vi "Draw Overlay.vi"(8 "error in (no error)":errorcluster, 11 "Terminal in":refnum<class "Terminal.lvclass">) -> (0 "error out":errorcluster, 3 "Terminal out":refnum<class "Terminal.lvclass">)   [LabVIEW 2020, in "Terminal.lvlib" / "Terminal.lvclass"]
uses:
  Terminal.lvclass
  Text Attributes.ctl
  Terminal.lvclass/Terminal.ctl
  <vilib>/IlluminatedG/lv-stream/Connection/Connection.lvclass
  Terminal.lvlib
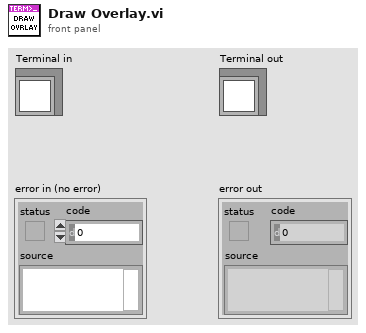
[diagram p1: front panel]
types:
  T1 = typedef "Terminal.lvlib/Text Attributes.ctl" = cluster{"FG":u32, "BG":u32, "Bold":bool, "Italic":bool, "Underline":bool, "Strike":bool, "Inverse":bool}
  T2 = typedef "Terminal.lvlib/Terminal.lvclass/Ref Data.ctl" = cluster{"Connection":refnum<class "Connection.lvclass">, "Read Loop Running":bool, "Parse State":T3, "Terminal Options":T7, "Font Metrics":T10, "Scroll":i32, "Close Read Loop":bool}
  T3 = typedef "Terminal.lvlib/Terminal.lvclass/Parse State.ctl" = cluster{"Buffer State":T4, "Cursor":T5, "Attributes":T1}
  T4 = typedef "Terminal.lvlib/Terminal.lvclass/Buffer State.ctl" = cluster{"Sequence":string, "ESC":bool, "Alt Buf":bool}
  T5 = typedef "Terminal.lvlib/Terminal.lvclass/Cursor.ctl" = cluster{"Cur":T6, "Saved":T6}
  T6 = typedef "Terminal.lvlib/Terminal.lvclass/Position.ctl" = cluster{"Row":i32, "Col":i32}
  T7 = typedef "Terminal.lvlib/Terminal Options.ctl" = cluster{"Implied CR with LF":bool, "Local Echo":bool, "Tab Width":i32, "Color Scheme":T8, "Default FG":T9, "Default BG":T9, "History Length":i32, "Font Face":string, "Font Size":i16, "Rows":i32, "Cols":i32}
  T8 = typedef "Terminal.lvlib/Color Scheme.ctl" = cluster{"Black":u32, "Red":u32, "Green":u32, "Yellow":u32, "Blue":u32, "Magenta":u32, "Cyan":u32, "White":u32, "Bright Black":u32, "Bright Red":u32, "Bright Green":u32, "Bright Yellow":u32, "Bright Blue":u32, "Bright Magenta":u32, "Bright Cyan":u32, "Bright White":u32}
  T9 = typedef "Terminal.lvlib/Color.ctl" = i8
  T10 = typedef "Terminal.lvlib/Terminal.lvclass/Font Metrics.ctl" = cluster{"Width":i16, "Height":i16}
  T11 = typedef "LVBoundsTypeDef.ctl" = cluster{"Width":u32, "Height":u32}
  T12 = cluster{"Font Name:":string, "Size":i16, "Strikeout?":bool, "Italic?":bool, "Underline?":bool, "Outline?":bool, "Shadow?":bool, "Bold?":bool}
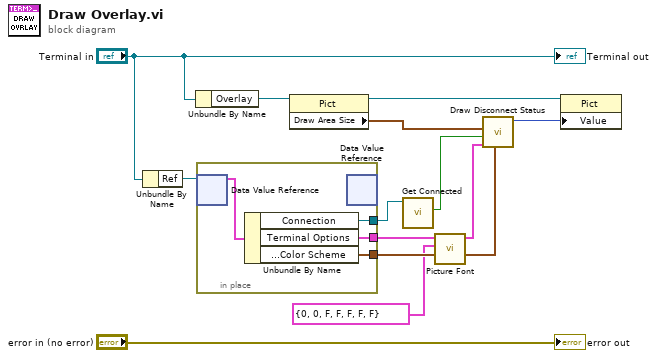
[diagram p0: block diagram]
diagram:
  n1 = Unbundle By Name("Terminal in") -> ("Ref"=w11:refnum<data-value>)
  n2 = Unbundle By Name("Terminal in") -> ("Overlay"=w12:refnum<vi>)
  n3 = in-place {
    in-place-border: [w16] -> w9
    in-place-border: [w15] -> w4
    in-place-border: [w14] -> w3
    n4 = in-place-dvr #1(w11) -> (w17:T2)  [unwired: 1 out]
    n5 = Unbundle By Name(w17) -> ("Connection"=w16:refnum<class "Connection.lvclass">, "Terminal Options"=w14:T7, "Terminal Options.Color Scheme"=w15:T8)
    n6 = in-place-dvr #1() -> ()  [unwired: 1 in, 2 out]
  }
  n7 = property class="Pict"(reference=w12) -> (reference out=w8:refnum<vi>, "Draw Area Size"=w7:T11)  [unwired: 1 in, 1 out]
  n8 = call <vilib>:"Get Connected.vi"("Connection in"=w9) -> ("Connected"=w6:bool)  [unwired: 8 in, 2 out]
  n9 = call "Picture Font.vi"("Text Attributes"=T1 {"FG"=0, "BG"=0, "Bold"=FALSE, "Italic"=FALSE, "Underline"=FALSE, "Strike"=FALSE, "Inverse"=FALSE}, "Terminal Options"=w3) -> ("Picture Font"=w1:T12)  [unwired: 6 in, 3 out]
  n10 = call "Draw Disconnect Status.vi"("Color Scheme"=w4, "Font"=w1, "Connected"=w6, "Draw Area Size"=w7) -> ("Picture"=w5:picture)  [unwired: 7 in]
  n11 = property class="Pict"(reference=w8, "Value"=w5) -> ()  [unwired: 1 in, 2 out]
  "error out" <- "error in (no error)"
  "Terminal out" <- "Terminal in"
